vi "Write TOC.vi"(0 "PDF Report Class in":refnum<class "PDF Report Class.lvclass">, 7 "TOC":T1={"Title"="Table of Contents", "Title Font"={"Name"="", "Size"=0.0, "Color"=0, "Style"={"Bold"=TRUE, "Italic"=FALSE, "Underline"=FALSE, "Strikeout"=FALSE}, "Type"={"Type&direction"=enum."Select", "Embedded"=FALSE, "Encoding"=""}}, "Chapter and section Font"={"Name"="", "Size"=-1.0, "Color"=0, "Style"={"Bold"=TRUE, "Italic"=FALSE, "Underline"=FALSE, "Strikeout"=FALSE}, "Type"={"Type&direction"=enum."Select", "Embedded"=FALSE, "Encoding"=""}}, "First TOC page"=0, "Add TOC?"=FALSE}, 11 "error in (no error)":errorcluster) -> (4 "PDF Report Class out":refnum<class "PDF Report Class.lvclass">, 15 "error out":errorcluster)   [LabVIEW 2019, in "Exaprom PDF.lvlib" / "PDF Report Class.lvclass"]
uses:
  PDF Report Class.lvclass
  Controls/Chapter Controls/TOC.ctl
  Controls/Font Controls/Font complete cluster.ctl
  Controls/Font Controls/Font size.ctl
  Controls/Font Controls/Font color.ctl
  Controls/Font Controls/Type and encoding.ctl
  Controls/Text Controls/Unicode/Type and run direction.ctl
  PDF Report Class.lvclass/PDF Report Class.ctl
  Exaprom PDF.lvlib
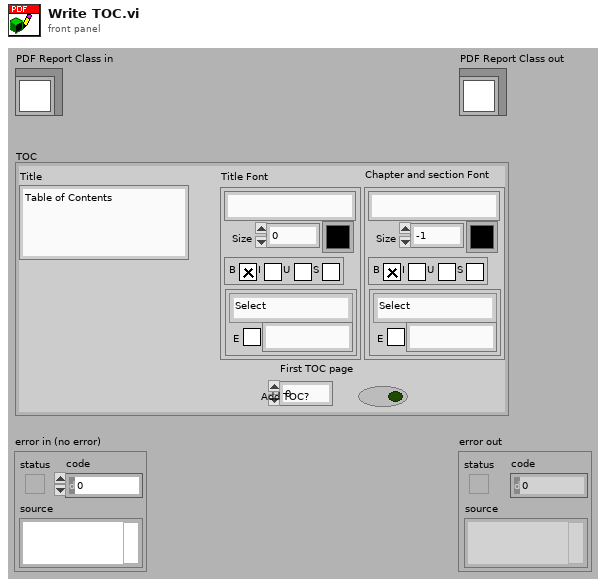
[diagram p1: front panel]
types:
  T1 = typedef "Exaprom PDF.lvlib/TOC.ctl" = cluster{"Title":string, "Title Font":T2, "Chapter and section Font":T2, "First TOC page":u16, "Add TOC?":bool}
  T2 = typedef "Exaprom PDF.lvlib/Font complete cluster.ctl" = cluster{"Name":string, "Size":T3, "Color":T4, "Style":cluster{"Bold":bool, "Italic":bool, "Underline":bool, "Strikeout":bool}, "Type":T5}
  T3 = typedef "Exaprom PDF.lvlib/Font size.ctl" = sgl
  T4 = typedef "Exaprom PDF.lvlib/Font color.ctl" = u32
  T5 = typedef "Exaprom PDF.lvlib/Type and encoding.ctl" = cluster{"Type&direction":T6, "Embedded":bool, "Encoding":string}
  T6 = typedef "Exaprom PDF.lvlib/Type and run direction.ctl" = enum16{"Select", "ASCII", "UTF-16", "UTF-16 (default)", "UTF-16 (LTR)", "UTF-16 (RTL)"}
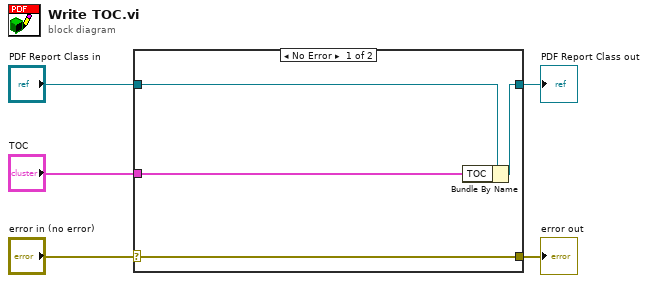
[diagram p0: block diagram]
diagram:
  n1 = case shown="No Error" "error in (no error)" {
    selector: "error in (no error)" -> [w9 w10]
    tunnel: [w9 w10] -> w4
    tunnel: [w7 w11] -> w2
    tunnel: "PDF Report Class in" -> [w8 w11]
    tunnel: "TOC" -> [w6 _]
    frame No Error {
      n2 = Bundle By Name(cluster=w8, "TOC"=w6) -> (w7:refnum<class "PDF Report Class.lvclass">)
    }
    frame Error {
    }
  }
  "error out" <- w4
  "PDF Report Class out" <- w2
